vi "Preview Vacuum State.vi"(8 "error in (no error)":errorcluster, 11 "Transfer Line in":refnum<class "Transfer Line.lvclass">) -> (0 "error out":errorcluster, 2 "Vacuum State":T1, 3 "Transfer Line out":refnum<class "Transfer Line.lvclass">)   [LabVIEW 2015, in "cRIO-Carbondioxide.lvlib" / "CO2-Actor.lvlib" / "Transfer Line.lvclass"]
uses:
  Transfer Line.lvclass
  Controls/Vacuum State Enumerator.ctl
  Transfer Line.lvclass/Transfer Line.ctl
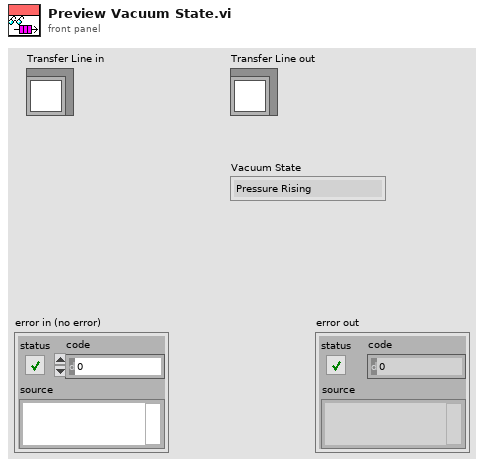
[diagram p1: front panel]
types:
  T1 = typedef "Vacuum State Enumerator.ctl" = enum16{"Pressure Rising", "Plateau", "Pressure Dropping", "Valley", "Low Valley", "Leak", "Unknown"}
  T2 = typedef "Vacuum State Cluster.ctl" = cluster{"Vacuum State":T1, "Pressure":dbl, "Raw Pressure":dbl, "d/dt":dbl}
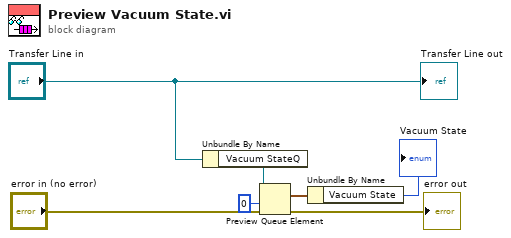
[diagram p0: block diagram]
diagram:
  n1 = Unbundle By Name("Transfer Line in") -> ("Vacuum StateQ"=w5:refnum<queue>)
  n2 = Preview Queue Element(queue=w5, timeout in ms (-1)=0, error in (no error)="error in (no error)") -> (element=w3:T2, error out=→"error out":errorcluster)  [unwired: 2 out]
  n3 = Unbundle By Name(w3) -> ("Vacuum State"=→"Vacuum State":T1)
  "Transfer Line out" <- "Transfer Line in"
